vi "Update.vi"(8 "error in (no error)":errorcluster, 10 "Angle Turned":dbl, 11 "TurnInstruction.lvclass":refnum<class "TurnInstruction.lvclass">) -> (0 "error out":errorcluster, 3 "TurnInstruction.lvclass 2":refnum<class "TurnInstruction.lvclass">)   [LabVIEW 2015, in "TurnInstruction.lvclass"]
uses:
  TurnInstruction.lvclass
  TurnInstruction.lvclass/TurnInstruction.ctl
panel:
  out "Remaining":dbl
  out "x-y":dbl
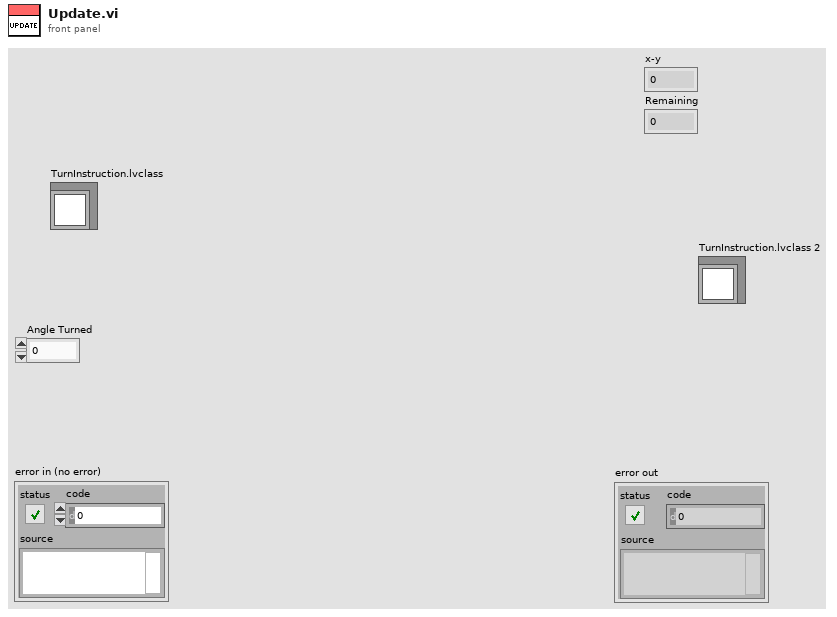
[diagram p1: front panel]
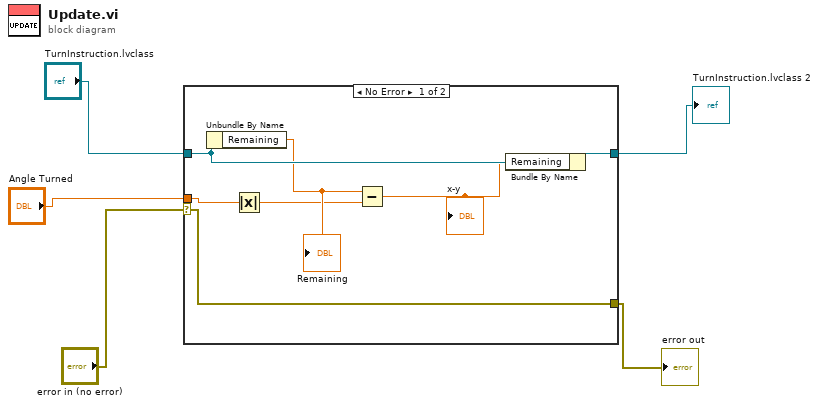
[diagram p0: block diagram]
diagram:
  n1 = case shown="No Error" "error in (no error)" {
    selector: "error in (no error)" -> [w12 w14]
    tunnel: [w12 w14] -> w4
    tunnel: [w10 w13] -> w3
    tunnel: "TurnInstruction.lvclass" -> [w11 w13]
    tunnel: "Angle Turned" -> [w7 _]
    frame No Error {
      n2 = Unbundle By Name(w11) -> ("Remaining"=w9:dbl)
      "Remaining" <- w9
      n3 = Absolute Value(x=w7) -> (abs(x)=w6:dbl)
      n4 = Subtract(x=w9, y=w6) -> (x-y=w8:dbl)
      "x-y" <- w8
      n5 = Bundle By Name(cluster=w11, "Remaining"=w8) -> (w10:refnum<class "TurnInstruction.lvclass">)
    }
    frame Error {
    }
  }
  "error out" <- w4
  "TurnInstruction.lvclass 2" <- w3
